vi "WriteConfig.vi"(0 "reference in":refnum<class "NeedleValve.lvclass">, 11 "error in (no error)":errorcluster) -> (4 "reference out":refnum<class "NeedleValve.lvclass">, 15 "error out":errorcluster)   [LabVIEW 2019, in "NeedleValve.lvclass"]
uses:
  NeedleValve.lvclass
  D:/GIT H4000/H4000/src/Device_class/Device.lvclass
  D:/GIT H4000/H4000/src/Proccess_class/Proccess.lvclass
  Proccess_class/Proccess.lvclass/Proccess.ctl
  Device_class/Device.lvclass/Device.ctl
  NeedleValve.lvclass/NeedleValve.ctl
  ConfigInterface_class/ConfigInterface.lvclass
  Proccess_class/Proccess.lvclass
  Device_class/Device.lvclass
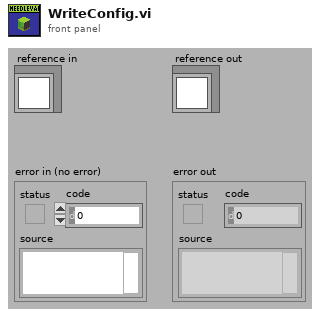
[diagram p1: front panel]
types:
  T1 = typedef "Proccess.lvclass/TAGs.ctl" = cluster{"TAG":string, "PTAG":string, "DESC":string}
  T2 = typedef "Needle Valve Settings.ctl" = cluster{"average size":i32, "open force":u16, "close force":u16, "open settings":T3, "close settings":T3, "Offset angle":dbl, "Start angle":dbl}
  T3 = typedef "MB_ENGINE.lvclass/Settings.ctl" = cluster{"ACC Steps Per Sec^2":u16, "DEC Steps Per Sec^2":u16, "Min Velosity Step Per Sec":u16, "Max Velosity Step Per Sec":u16, "MicroStep":u16}
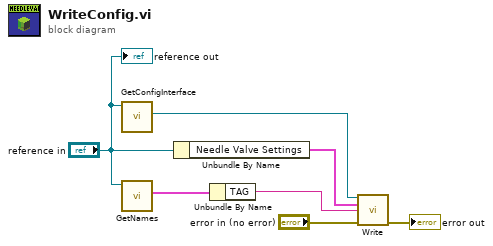
[diagram p0: block diagram]
diagram:
  n1 = call "GetConfigInterface.vi"("Device in"="reference in") -> ("ConfigInterface"=w5:refnum<class "ConfigInterface.lvclass">)  [unwired: 10 in]
  n2 = call "GetNames.vi"("Proccess in"="reference in") -> ("Tags"=w6:T1)  [unwired: 10 in]
  n3 = Unbundle By Name("reference in") -> ("Needle Valve Settings"=w7:T2)
  n4 = Unbundle By Name(w6) -> ("TAG"=w1:string)
  n5 = call-dynamic "Write.vi"("reference in"=w5, "Data"=w7, "Name"=w1, "error in (no error)"="error in (no error)") -> ("error out"=→"error out":errorcluster)  [unwired: 8 in, 3 out]
  "reference out" <- "reference in"
